vi "ReadConfig.vi"(0 "SharedVariableWrapper in":refnum<class "SharedVariableWrapper.lvclass">, 11 "error in":errorcluster) -> (4 "SharedVariableWrapper":refnum<class "SharedVariableWrapper.lvclass">, 6 "config":T1, 15 "error out":errorcluster)   [LabVIEW 2019, in "SharedVariableWrapper.lvclass"]
uses:
  SharedVariableWrapper.lvclass
  Config.ctl
  SharedVariableWrapper.lvclass/SharedVariableWrapper.ctl
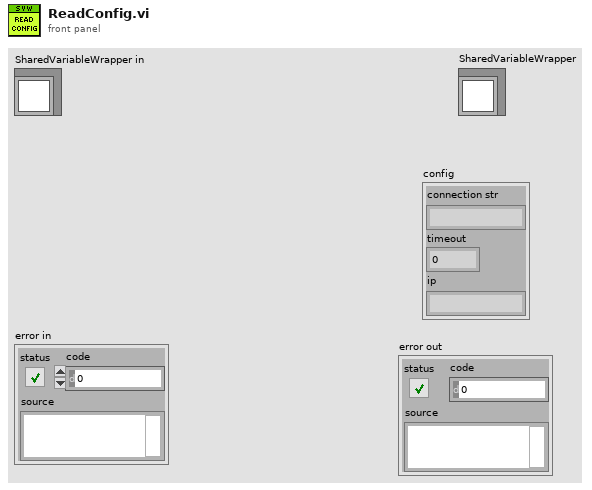
[diagram p1: front panel]
types:
  T1 = typedef "SharedVariableWrapper.lvclass/Config.ctl" = cluster{"connection str":string, "timeout":dbl, "ip":string}
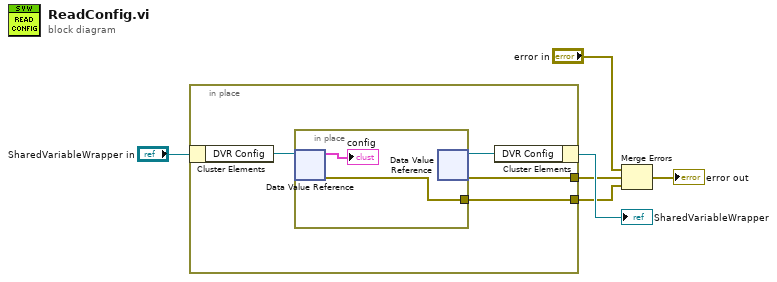
[diagram p0: block diagram]
diagram:
  n1 = in-place {
    in-place-border: [w8] -> w4
    in-place-border: [w7] -> w3
    n2 = in-place-cluster #1("SharedVariableWrapper in") -> ("DVR Config"=w10:refnum<data-value>)
    n3 = in-place {
      in-place-border: [w12] -> w7
      n4 = in-place-dvr #2(w10) -> (→"config":T1, w12:errorcluster)
      n5 = in-place-dvr #2() -> (w9:refnum<data-value>, w8:errorcluster)  [unwired: 1 in]
    }
    n6 = in-place-cluster #1("DVR Config"=w9) -> (→"SharedVariableWrapper":refnum<class "SharedVariableWrapper.lvclass">)
  }
  n7 = Merge Errors("error in", w4, w3) -> (→"error out":errorcluster)
